vi "Connect.vi"(8 "error in (no error)":errorcluster, 9 "Custom Connection Data":variant, 10 "Connection Name":string, 11 "CIFTag in":refnum<class "CIFTag.lvclass">) -> (0 "error out":errorcluster, 3 "CIFTag out":refnum<class "CIFTag.lvclass">)   [LabVIEW 2021, in "CIFTag.lvclass"]
uses:
  CIFTag.lvclass
  CIFTag.lvclass/CIFTag.ctl
  CIFUtilities/CIFChannels/CIFChannels.lvclass
  <vilib>/CIFChannels/CIFChannelCore.lvlib
  CIFUtilities/CIFChannels/Typedef/Channel State.ctl
  D:/dev/CIF-LVCore/src/CIFUtilities/CIFChannels/CIFChannels.lvclass
  D:/dev/CIF-LVCore/src/Channels/CIFTag/CIFTag/CIFTag.lvclass
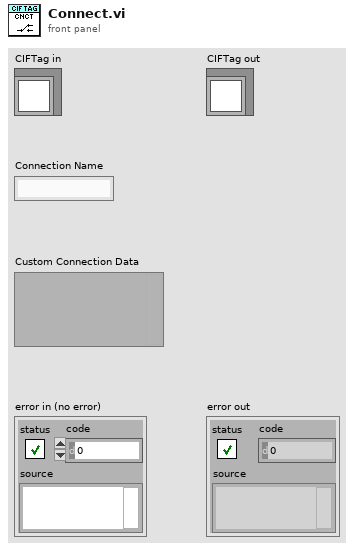
[diagram p1: front panel]
types:
  T1 = typedef "CIFChannels.lvclass/Channel State.ctl" = enum16{"Creating", "Disconnected", "Connecting", "Connected", "Destroying"}
  T2 = typedef "CIFChannels.lvclass/Direction.ctl" = enum16{"Publisher", "Subscriber"}
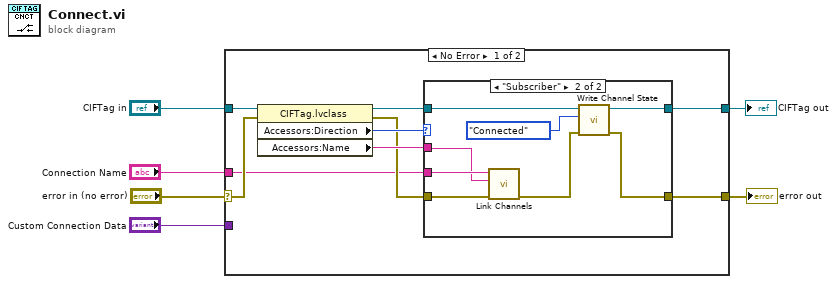
[diagram p0: block diagram]
diagram:
  n1 = case shown="No Error" "error in (no error)" {
    selector: "error in (no error)" -> [w14 w27]
    tunnel: [w7 w27] -> w5
    tunnel: [w11 w26] -> w3
    tunnel: "CIFTag in" -> [w15 w26]
    tunnel: "Connection Name" -> [w8 _]
    tunnel: "Custom Connection Data" -> [_ _]
    frame No Error {
      n2 = property class="CIFTag.lvclass"(reference=w15, error in=w14) -> (reference out=w13:refnum<class "CIFTag.lvclass">, error out=w9:errorcluster, "Accessors:Direction"=w12:T2, "Accessors:Name"=w10:string)
      n3 = case shown="\"Subscriber\"" w12 {
        tunnel: w13 -> [w17 w25]
        tunnel: [w17 w19] -> w11
        tunnel: w10 -> [_ w23]
        tunnel: w9 -> [w16 w22]
        tunnel: w8 -> [_ w24]
        tunnel: [w16 w20] -> w7
        frame "Publisher" {
        }
        frame "Subscriber" {
          n4 = call <vilib>:"Link Channels.vi"("error in"=w22, "Consumer Channel Name"=w23, "Producer Channel Name"=w24) -> ("error out"=w21:errorcluster)  [unwired: 8 in]
          n5 = call "Write Channel State.vi"("error in (no error)"=w21, "Channel State"=Channel_State."Connected", "CIFChannels in"=w25) -> ("error out"=w20:errorcluster, "CIFChannels out"=w19:refnum<class "CIFTag.lvclass">)  [unwired: 7 in]
        }
      }
    }
    frame Error {
    }
  }
  "error out" <- w5
  "CIFTag out" <- w3
